vi "Localize Path.vi"(1 "Path":path) -> (0 "Local path":path)   [LabVIEW 2019]
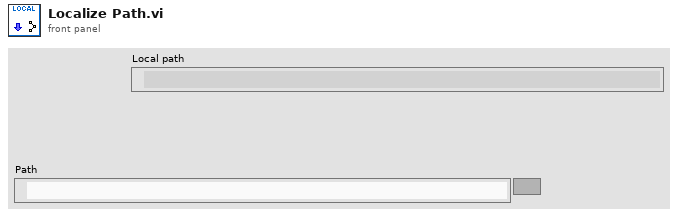
[diagram p1: front panel]
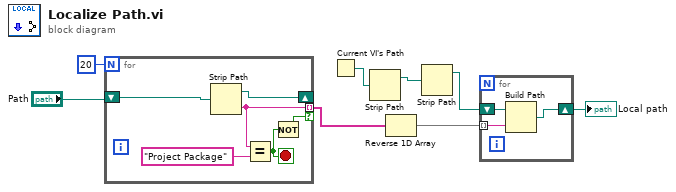
[diagram p0: block diagram]
diagram:
  n1 = for {
    N: 20 -> [_]
    shift-right: [w13] -> _
    shift-left: "Path" -> [w14]
    tunnel: [w12] -> w2 mode=indexing if=w9
    stop <- w10 stop-if-true
    n2 = Strip Path(path=w14) -> (stripped path=w13:path, name=w12:string)
    n3 = Equal?(x=w12, y="Project Package") -> (x = y?=w10:bool)
    n4 = Not(x=w10) -> (.not. x?=w9:bool)
  }
  n5 = Current VI's Path() -> (path=w4:path)
  n6 = Strip Path(path=w4) -> (stripped path=w5:path)  [unwired: 1 out]
  n7 = Reverse 1D Array(array=w2) -> (reversed array=w1:string[])
  n8 = Strip Path(path=w5) -> (stripped path=w6:path)  [unwired: 1 out]
  n9 = for {
    shift-right: [w15] -> w7
    shift-left: w6 -> [w17]
    tunnel: w1 -> [w16] mode=indexing
    n10 = Build Path(base path=w17, name or relative path=w16) -> (appended path=w15:path)
  }
  "Local path" <- w7
